vi "to string.vi"(8 "error in":errorcluster, 11 "module configuration in":refnum<class "fixed channel tag bus module configuration.lvclass">) -> (0 "error out":errorcluster, 1 "data":string, 2 "version":string, 3 "module configuration out":refnum<class "fixed channel tag bus module configuration.lvclass">)   [LabVIEW 2013, in "fixed channel tag bus module configuration.lvclass"]
doc: "Provides an interface for saving a module configuration to a file or other serialized data source. It is recommended that all children of this class store data in two sets--data required for its own initialization, and any data required for parent initialization--and that each implementation uses the <b>Call Parent Method</b> primitive to serialize parent information.\nNI Tag Bus Module Framework 1.0.3.43\nNI Systems Engineering"
uses:
  fixed channel tag bus module configuration.lvclass
  <vilib>/NI/Tag Bus Module Framework/module configuration/TBM module configuration.lvclass
  fixed channel tag bus module configuration.lvclass/fixed channel tag bus module configuration.ctl
  <vilib>/NI/Tag Bus/tag/tag descriptor.lvclass/tag descriptor.ctl
  <vilib>/NI/Tag Bus Module Framework/channel/TBM channel.lvclass
  <vilib>/NI/Tag Bus Module Framework/root configuration/TBM configuration.lvclass
  <vilib>/NI/Tag Bus/tag/tag descriptor.lvclass
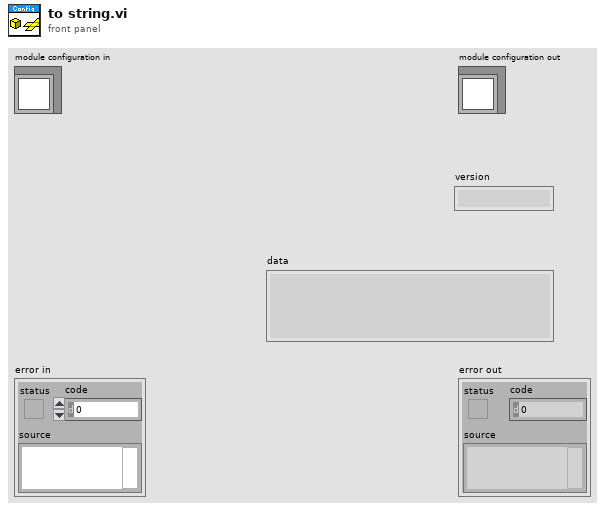
[diagram p1: front panel]
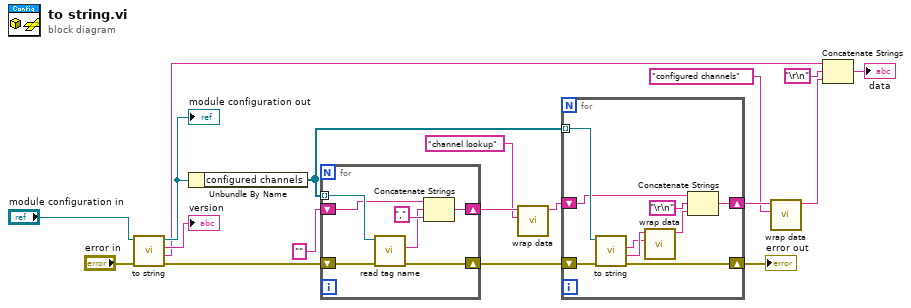
[diagram p0: block diagram]
diagram:
  n1 = call-parent "to string.vi"("error in"="error in", "module configuration in"="module configuration in") -> ("error out"=w12:errorcluster, "data"=w8:string, "version"=→"version":string, "module configuration out"=w15:refnum<class "fixed channel tag bus module configuration.lvclass">)  [unwired: 6 in]
  "module configuration out" <- w15
  n2 = Unbundle By Name(w15) -> ("configured channels"=w9:refnum<class "TBM channel.lvclass">[])
  n3 = for {
    tunnel: w9 -> [w25] mode=indexing
    shift-right: [w23] -> w11
    shift-left: w12 -> [w24]
    shift-right: [w21] -> w3
    shift-left: "" -> [w22]
    n4 = call <vilib>:"read tag name.vi"("error in"=w24, "system tag in"=w25) -> ("error out"=w23:errorcluster, "name"=w19:string)  [unwired: 7 in, 1 out]
    n5 = Concatenate Strings(w22, w19, "," ("string")) -> (w21:string)
  }
  n6 = call <vilib>:"wrap data.vi"("identifier"="channel lookup", "data to wrap"=w3) -> ("wrapped data"=w1:string)  [unwired: 9 in]
  n7 = for {
    tunnel: w9 -> [w34] mode=indexing
    shift-right: [w30] -> w14
    shift-left: w1 -> [w31]
    shift-right: [w28] -> w10
    shift-left: w11 -> [w29]
    n8 = call-dynamic "to string.vi"("error in"=w29, "channel in"=w34) -> ("error out"=w28:errorcluster, "channel data"=w33:string, "identifier"=w32:string)  [unwired: 6 in, 1 out]
    n9 = call <vilib>:"wrap data.vi"("identifier"=w32, "data to wrap"=w33) -> ("wrapped data"=w26:string)  [unwired: 9 in]
    n10 = Concatenate Strings(w31, "\r\n", w26) -> (w30:string)
  }
  "error out" <- w10
  n11 = call <vilib>:"wrap data.vi"("identifier"="configured channels", "data to wrap"=w14) -> ("wrapped data"=w7:string)  [unwired: 9 in]
  n12 = Concatenate Strings(w8, "\r\n", w7) -> (→"data":string)
